vi "Diagnostic Cycle.vi"(8 "error in (no error)":errorcluster, 11 "MSX-E3701 in":refnum<class "MSX-E3701.lvclass">) -> (0 "error out":errorcluster, 3 "MSX-E3701 out":refnum<class "MSX-E3701.lvclass">)   [LabVIEW 2014, in "MSX-E3701.lvlib" / "MSX-E3701.lvclass"]
doc: "Toma una Cantidad de muestras definidas Diagnostic Data. Muestras Diag. Cycle y las promedia."
uses:
  MSX-E3701.lvclass
  MSX-E3701.lvclass/MSX-E3701.ctl
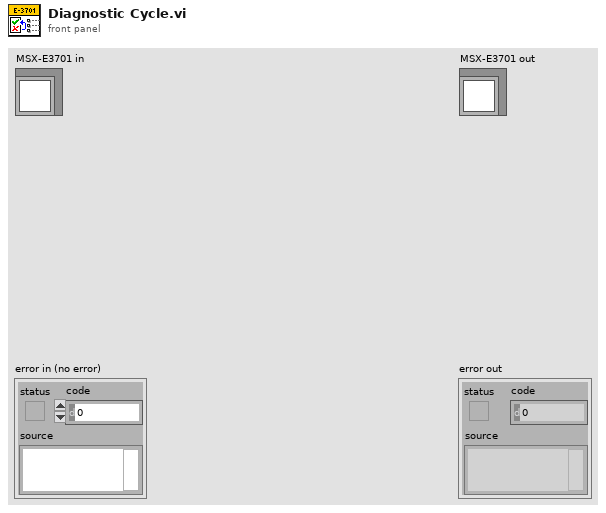
[diagram p1: front panel]
types:
  T1 = typedef "DriverMasterSync.lvlibp/WINFAS 2 Data Queue.lvlib/Acquisition Data 1 Sample Cluster.ctl" = cluster{"TDX":sgl[], "Encoder":sgl}
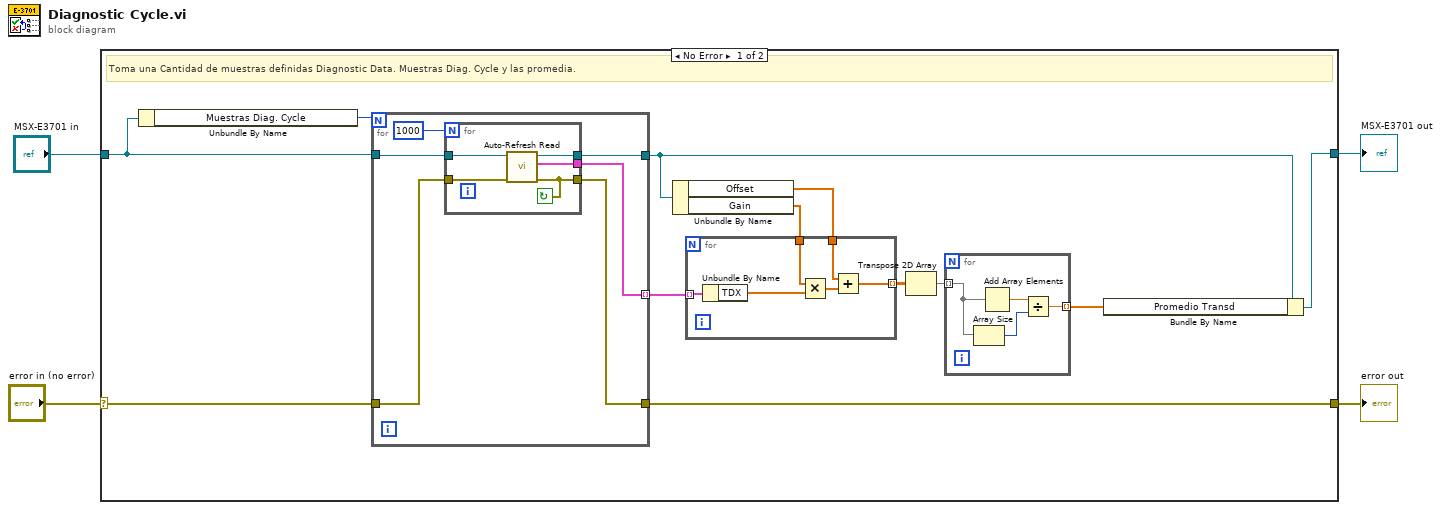
[diagram p0: block diagram]
diagram:
  n1 = case shown="No Error" "error in (no error)" {
    selector: "error in (no error)" -> [w16 w38]
    tunnel: [w12 w38] -> w1
    tunnel: [w15 w39] -> w2
    tunnel: "MSX-E3701 in" -> [w9 w39]
    frame No Error {
      # "Toma una Cantidad de muestras definidas Diagnostic Data. Muestras Diag. Cycle y las promedia."
      n2 = Unbundle By Name(w9) -> ("Muestras Diag. Cycle"=w8:u32)
      n3 = for {
        N: w8 -> [_]
        tunnel: [w19] -> w14 mode=indexing
        tunnel: w9 -> [w17]
        tunnel: [w20] -> w7
        tunnel: w16 -> [w22]
        tunnel: [w18] -> w12
        n4 = for {
          N: 1000 -> [_]
          tunnel: w22 -> [w25]
          tunnel: w17 -> [w27]
          tunnel: [w26] -> w20
          tunnel: [w24] -> w18
          tunnel: [w23] -> w19
          stop <- w24 continue-if-true
          n5 = call-dynamic "Auto-Refresh Read.vi"("error in (no error)"=w25, "MSX-E3701 in"=w27) -> ("error out"=w24:errorcluster, "1 Sample"=w23:T1, "MSX-E3701 out"=w26:refnum<class "MSX-E3701.lvclass">)  [unwired: 6 in, 1 out]
        }
      }
      n6 = Unbundle By Name(w7) -> ("Offset"=w5:sgl[], "Gain"=w6:sgl[])
      n7 = for {
        tunnel: w14 -> [w37] mode=indexing
        tunnel: [w35] -> w11 mode=indexing
        tunnel: w6 -> [w33]
        tunnel: w5 -> [w32]
        n8 = Unbundle By Name(w37) -> ("TDX"=w34:sgl[])
        n9 = Multiply(x=w33, y=w34) -> (x*y=w36:sgl[])
        n10 = Add(x=w32, y=w36) -> (x+y=w35:sgl[])
      }
      n11 = Transpose 2D Array(2D array=w11) -> (transposed array=w10:sgl[][])
      n12 = for {
        tunnel: w10 -> [w31] mode=indexing
        tunnel: [w28] -> w13 mode=indexing
        n13 = Array Size(array=w31) -> (size(s)=w30:i32)
        n14 = Add Array Elements(numeric array=w31) -> (sum=w29:sgl)
        n15 = Divide(x=w29, y=w30) -> (x/y=w28:sgl)
      }
      n16 = Bundle By Name(cluster=w7, "Promedio Transd"=w13) -> (w15:refnum<class "MSX-E3701.lvclass">)
    }
    frame Error {
    }
  }
  "error out" <- w1
  "MSX-E3701 out" <- w2
